vi "周期参数设置.vi"(11 "测量参数输入":T1) -> (2 "数组":string[][](array[string]), 3 "输出":bool)   [LabVIEW 2016, in "TimingControl.lvlib" / "TimingControl.lvclass"]
uses:
  TimingControl.lvclass
  <vilib>/Utility/miscctls.llb/LVPointTypeDef.ctl
panel:
  in  "启动命令":T2 caption="00：00"
  in  "周期模式":T3
  in  "每日启动":T4
  in  "保存":bool
  in  "退出":bool
  in  "每月启动":T5
  in  "每周启动":T6
  out "周期模式选择卡":enum32{"选项卡 1", "选项卡 2"}(tab)
  in  "定点周期":T7 {"时间" items=["00:00", "01:00", "02:00", "03:00", "04:00", "05:00", "06:00", "07:00", "08:00", "09:00", "10:00", "11:00", "12:00", "13:00", "14:00", "15:00", "16:00", "17:00", "18:00", "19:00", "20:00", "21:00", "22:00", "23:00"]}
  in  "间隔启动 2":T8
  in  "测量参数":string(combo)
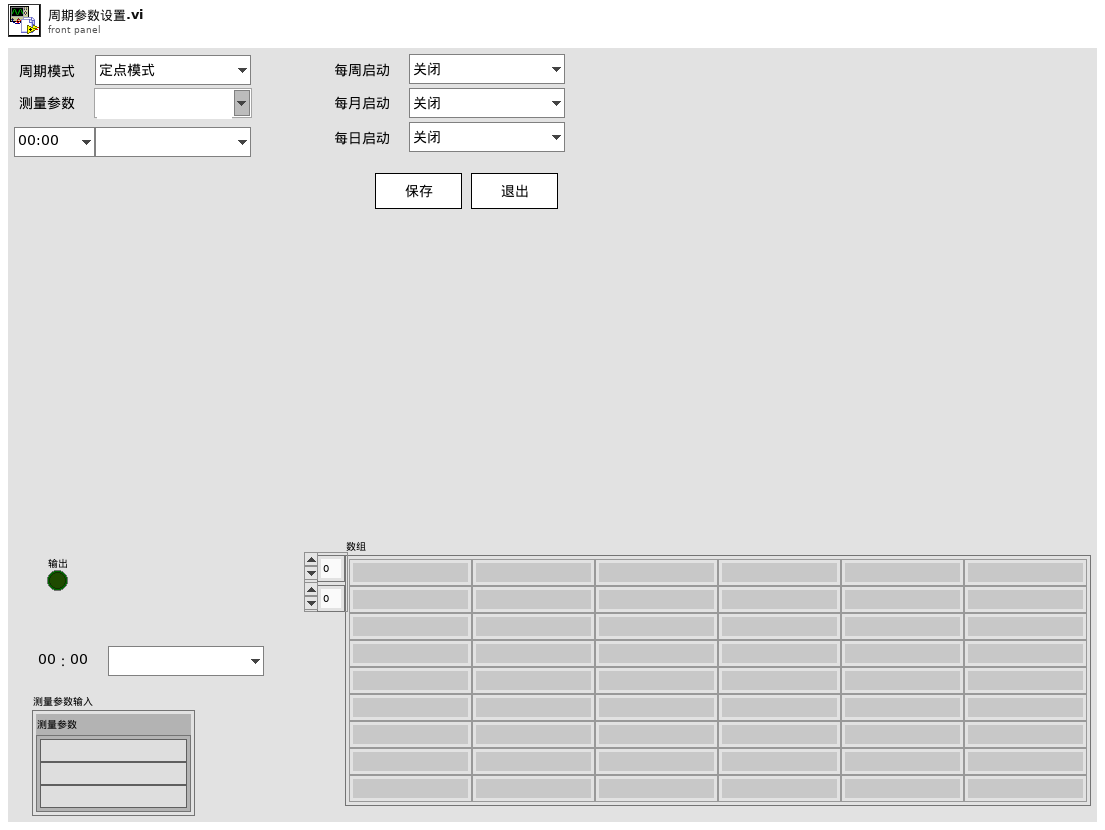
[diagram p1: front panel]
types:
  T1 = typedef "TimingControl.lvlib/TimingControl.lvclass/测量参数.ctl" = cluster{"测量参数":string[]}
  T2 = typedef "TimingControl.lvlib/TimingControl.lvclass/启动命令选择.ctl" = enum16{"", "水样测试", "标样核查", "零点核查", "跨度核查", "空白测试", "平行样测试", "加标回收", "空白校准", "标样校准", "初始化(清洗)"}
  T3 = typedef "TimingControl.lvlib/TimingControl.lvclass/周期模式设置.ctl" = enum16{"定点模式", "间隔模式"}
  T4 = typedef "TimingControl.lvlib/TimingControl.lvclass/每日启动.ctl" = enum16{"关闭", "每日"}
  T5 = typedef "TimingControl.lvlib/TimingControl.lvclass/每月启动.ctl" = enum16{"关闭", "1号", "2号", "3号", "4号", "5号", "6号", "7号", "8号", "9号", "10号", "11号", "12号", "13号", "14号", "15号", "16号", "17号", "18号", "19号", "20号", "21号", "22号", "23号", "24号", "25号", "26号", "27号", "28号", "29号", "30号", "31号"}
  T6 = typedef "TimingControl.lvlib/TimingControl.lvclass/每周启动.ctl" = enum16{"关闭", "周日", "周一", "周二", "周三", "周四", "周五", "周六"}
  T7 = typedef "TimingControl.lvlib/TimingControl.lvclass/定点周期设置.ctl" = cluster{"时间":u16, "启动命令":T2}
  T8 = typedef "TimingControl.lvlib/TimingControl.lvclass/间隔启动设置.ctl" = cluster{"启动命令":T2, "启动间隔":dbl, "启动次数":i32}
  T9 = typedef "LVPointTypeDef.ctl" = cluster{"Horizontal":i16, "Vertical":i16}
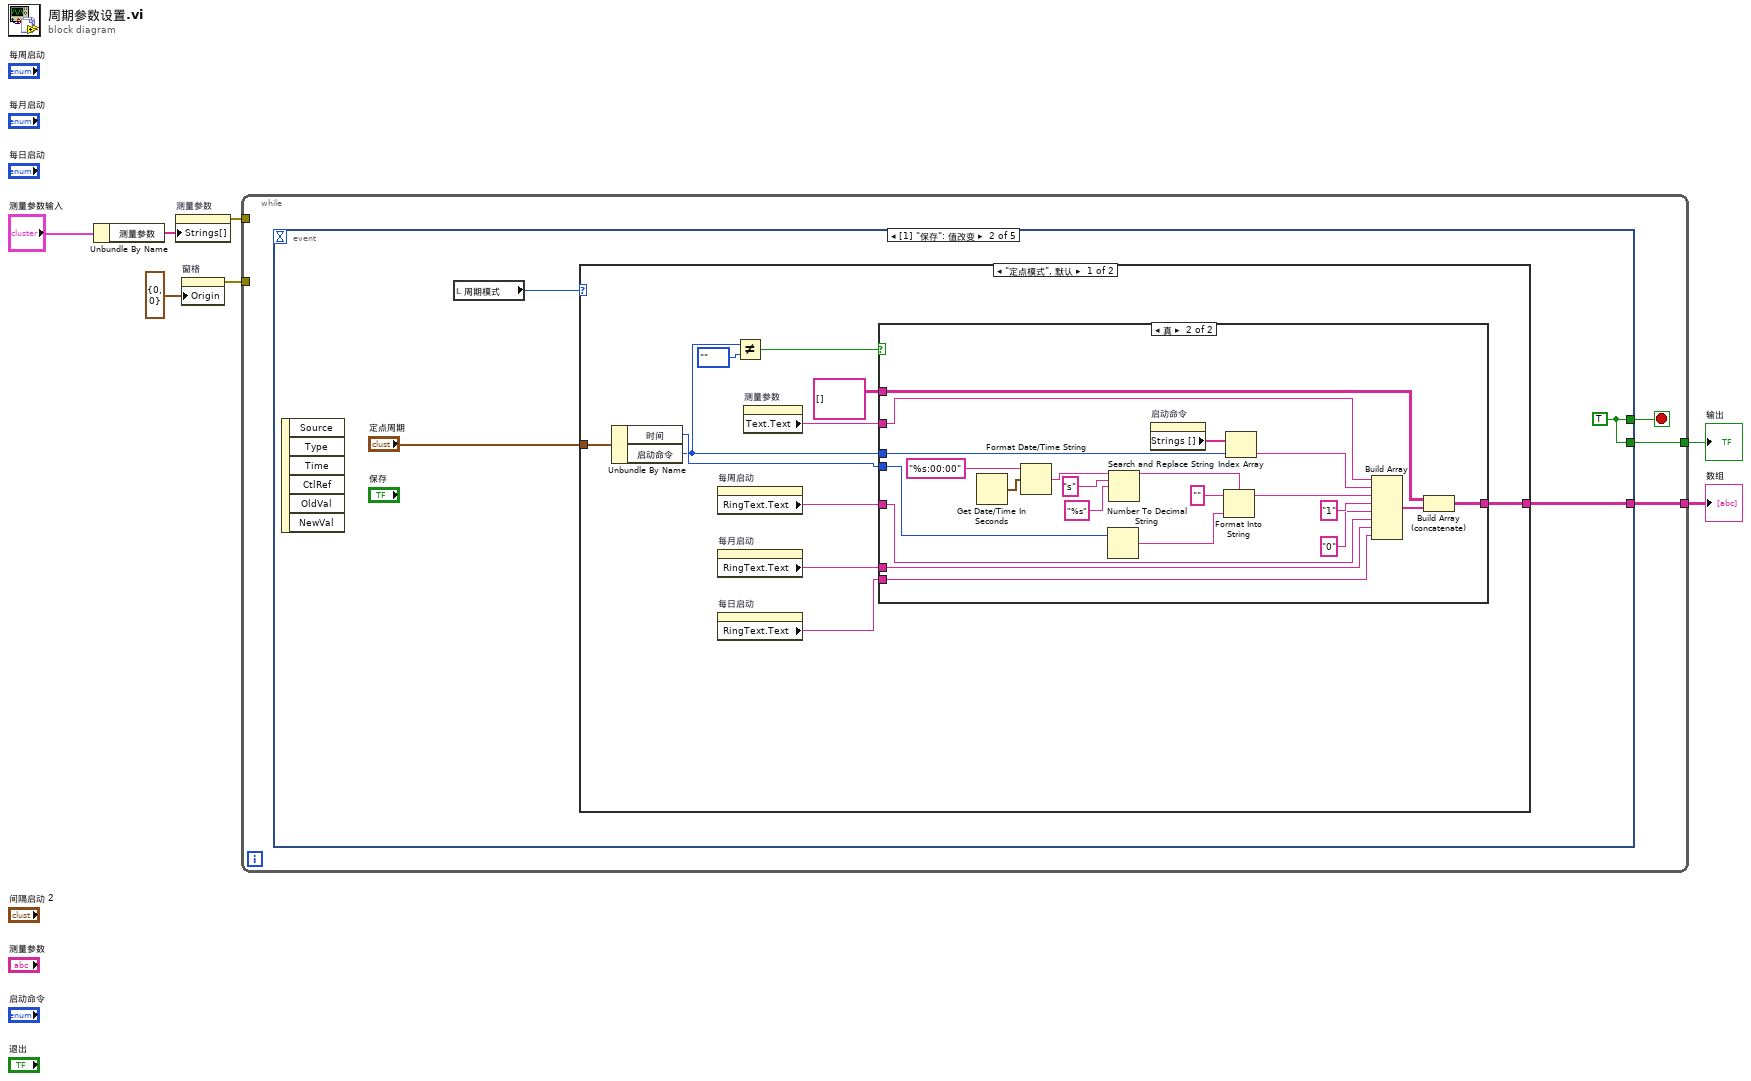
[diagram p0: block diagram]
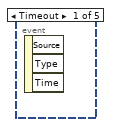
[diagram p2: hidden frame]
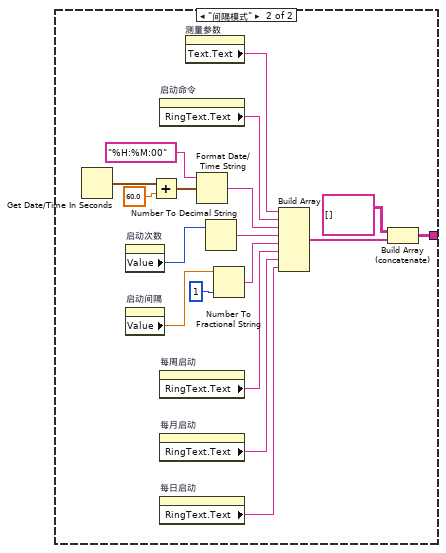
[diagram p4: hidden frame]
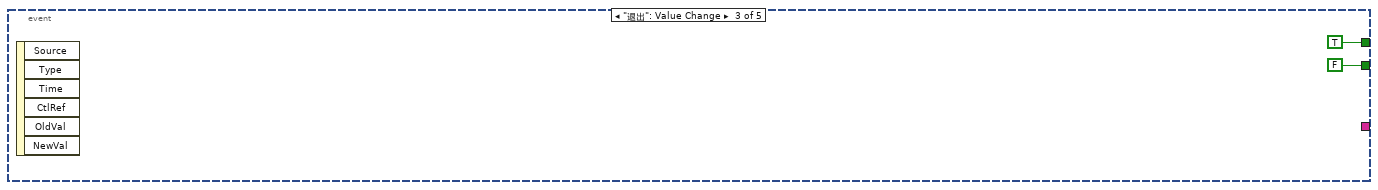
[diagram p5: hidden frame]
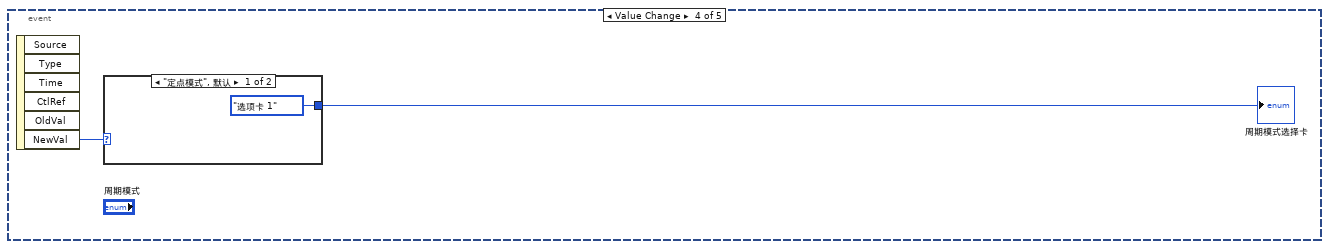
[diagram p6: hidden frame]
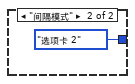
[diagram p7: hidden frame]
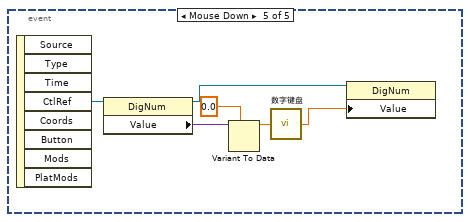
[diagram p8: hidden frame]
diagram:
  n1 = Unbundle By Name("测量参数输入") -> ("测量参数"=w1:string[])
  n2 = property on="测量参数" class="CmbBox"("Strings[]"=w1) -> (error out=w3:errorcluster)  [unwired: 2 in, 1 out]
  n3 = property on="窗格" class="Pane"("Origin"=T9 {"Horizontal"=0, "Vertical"=0} ("原点")) -> (error out=w4:errorcluster)  [unwired: 2 in, 1 out]
  n4 = while {
    tunnel: [w9] -> w7
    tunnel: [w8] -> w6
    tunnel: w4 -> [_]
    tunnel: w3 -> [_]
    stop <- w10 stop-if-true
    n5 = event shown="[1] \"保存\": 值改变" {
      selector: _ -> [_ _ _ _ _]
      dyn-events: _ -> [_ _ _ _ _]
      timeout: _ -> [_ _ _ _ _]
      tunnel: [_ w14 TRUE _ _] -> w10
      tunnel: [_ w14 FALSE _ _] -> w9
      tunnel: [_ w13 _ _ _] -> w8
      event Timeout {
        n6 = event-data() -> ()  [unwired: 1 in, 3 out]
      }
      event "保存": Value Change {
        w14 = TRUE
        n7 = event-data() -> ()  [unwired: 1 in, 6 out]
        n8 = local read "周期模式"() -> (w12:T3)
        n9 = case shown="\"定点模式\", 默认" w12 {
          tunnel: [w24 w65] -> w13
          tunnel: "定点周期" -> [w17 _]
          frame "定点模式", Default {
            n10 = Unbundle By Name(w17) -> ("时间"=w16:u16, "启动命令"=w15:T2)
            n11 = property on="每周启动" class="Enum (严格)"() -> ("RingText.Text"=w20:string)  [unwired: 2 in, 2 out]
            n12 = property on="每月启动" class="Enum (严格)"() -> ("RingText.Text"=w19:string)  [unwired: 2 in, 2 out]
            n13 = property on="每日启动" class="Enum (严格)"() -> ("RingText.Text"=w18:string)  [unwired: 2 in, 2 out]
            n14 = Not Equal?(x=w15, y=启动命令选择."") -> (x != y?=w22:bool)
            n15 = property on="测量参数" class="CmbBox"() -> ("Text.Text"=w21:string)  [unwired: 2 in, 2 out]
            n16 = case shown="真" w22 {
              tunnel: w15 -> [_ w47]
              tunnel: w21 -> [_ w45]
              tunnel: w20 -> [_ w44]
              tunnel: w19 -> [_ w43]
              tunnel: w18 -> [_ w42]
              tunnel: [w26 w39] -> w24
              tunnel: string[][] [] -> [w26 w41]
              tunnel: w16 -> [_ w38]
              frame False {
              }
              frame True {
                n17 = Get Date/Time In Seconds() -> (seconds since 1Jan1904=w36:timestamp)
                n18 = Format Date/Time String(time format string (%c)="%s:00:00" ("时间格式字符串(%c)"), seconds (now)=w36) -> (date/time string=w31:string)  [unwired: 1 in]
                n19 = Number To Decimal String(number=w38) -> (decimal integer string=w34:string)  [unwired: 1 in]
                n20 = Search and Replace String(input string=w31, search string="s" ("搜索字符串"), replace string="%s" ("替换字符串(\"\")")) -> (result string=w32:string)  [unwired: 5 in, 3 out]
                n21 = property on="启动命令" class="Enum (严格)"() -> ("Strings []"=w48:string[])  [unwired: 2 in, 2 out]
                n22 = Format Into String(format string=w32, initial string="" ("初始字符串"), w34) -> (resulting string=w33:string)  [unwired: 1 in, 1 out]
                n23 = Index Array(array=w48, index=w47) -> (element=w46:string)
                n24 = Build Array(w45, w46, w33, "1" ("元素"), "0" ("元素"), w44, w43, w42) -> (w40:string[])
                n25 = Build Array (concatenate)(w41, w40) -> (w39:string[][])
              }
            }
          }
          frame "间隔模式" {
            n26 = Get Date/Time In Seconds() -> (seconds since 1Jan1904=w56:timestamp)
            n27 = property on="启动次数" class="DigNum (严格)"() -> ("Value"=w53:i32)  [unwired: 2 in, 2 out]
            n28 = property on="启动间隔" class="DigNum (严格)"() -> ("Value"=w55:dbl)  [unwired: 2 in, 2 out]
            n29 = Add(x=w56, y=60.0) -> (x+y=w50:timestamp)
            n30 = property on="启动命令" class="Enum (严格)"() -> ("RingText.Text"=w63:string)  [unwired: 2 in, 2 out]
            n31 = property on="每周启动" class="Enum (严格)"() -> ("RingText.Text"=w60:string)  [unwired: 2 in, 2 out]
            n32 = property on="每月启动" class="Enum (严格)"() -> ("RingText.Text"=w59:string)  [unwired: 2 in, 2 out]
            n33 = property on="每日启动" class="Enum (严格)"() -> ("RingText.Text"=w58:string)  [unwired: 2 in, 2 out]
            n34 = property on="测量参数" class="CmbBox"() -> ("Text.Text"=w64:string)  [unwired: 2 in, 2 out]
            n35 = Format Date/Time String(time format string (%c)="%H:%M:00" ("时间格式字符串(%c)"), seconds (now)=w50) -> (date/time string=w61:string)  [unwired: 1 in]
            n36 = Number To Decimal String(number=w53) -> (decimal integer string=w52:string)  [unwired: 1 in]
            n37 = Number To Fractional String(number=w55, precision (6)=i16 1 ("精度(6)")) -> (F-format string=w54:string)  [unwired: 2 in]
            n38 = Build Array(w64, w63, w61, w52, w54, w60, w59, w58) -> (w57:string[])
            n39 = Build Array (concatenate)(string[][] [], w57) -> (w65:string[][])
          }
        }
      }
      event "退出": Value Change {
        n40 = event-data() -> ()  [unwired: 1 in, 6 out]
      }
      event Value Change {
        n41 = event-data() -> ("NewVal"=w70:T3)  [unwired: 1 in, 5 out]
        n42 = case shown="\"定点模式\", 默认" w70 {
          tunnel: [enum32{"选项卡 1", "选项卡 2"}."选项卡 1" ("周期模式选择卡") enum32{"选项卡 1", "选项卡 2"}."选项卡 2" ("周期模式选择卡")] -> w69
          frame "定点模式", Default {
          }
          frame "间隔模式" {
          }
        }
        "周期模式选择卡" <- w69
      }
      event Mouse Down {
        n43 = event-data() -> ("CtlRef"=w78:refnum<vi>)  [unwired: 1 in, 7 out]
        n44 = property class="DigNum"(reference=w78) -> (reference out=w74:refnum<vi>, "Value"=w76:variant)  [unwired: 1 in, 1 out]
        n45 = Variant To Data(type=0.0, Variant=w76) -> (data=w75:dbl)  [unwired: 1 in, 1 out]
        n46 = call "数字键盘.vi"("OldNumber"=w75) -> ("NewNumber"=w73:sgl)
        n47 = property class="DigNum"(reference=w74, "Value"=w73) -> ()  [unwired: 1 in, 2 out]
      }
    }
  }
  "输出" <- w7
  "数组" <- w6
